vi "Alarm Flir-Ax8.vi"() -> ()   [LabVIEW 2016]
uses:
  <vilib>/sound2/lvsound2.llb/Sampling Mode.ctl
  <vilib>/sound2/lvsound2.llb/Sound File Info (path).vi
  <vilib>/sound2/lvsound2.llb/Sound File Read Open.vi
  Global Flir-Ax8.vi
  <vilib>/sound2/lvsound2.llb/Sound File Read (DBL).vi
  <vilib>/sound2/lvsound2.llb/Sound Output Write (DBL).vi
panel:
  in  "Number of Samples/Iteration":i32=2500
  in  "Device ID":u32
  out "Current Iteration":i32
  out "Current Data":waveform(dbl)[](graph)
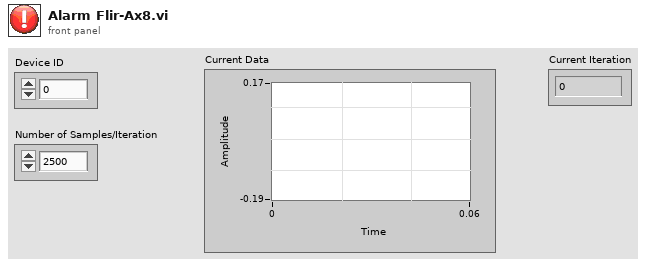
[diagram p1: front panel]
types:
  T1 = typedef "Sampling Mode.ctl" = i32
  T2 = typedef "Sound Data Format.ctl" = cluster{"sample rate (S/s)":dbl, "number of channels":i32, "bits per sample":i32}
  T3 = typedef "Sound File Refnum.ctl" = refnum<file>
  T4 = typedef "Sound Output Task ID.ctl" = u32
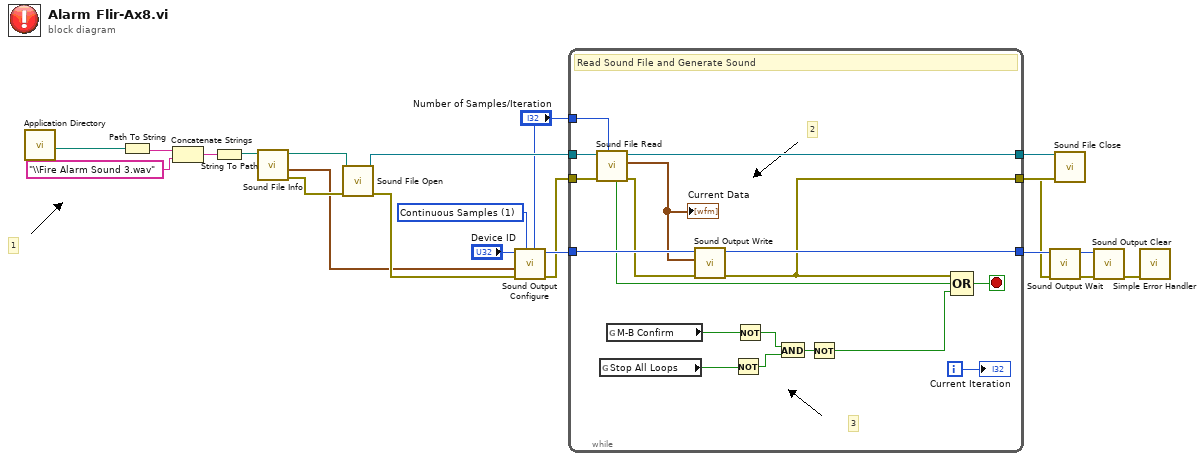
[diagram p0: block diagram]
diagram:
  w7 = T1 1 items=["Finite Samples", "Continuous Samples"] ("sample mode")
  # "1"
  n1 = call <vilib>:"Application Directory.vi"() -> ("Application Directory"=w2:path)
  n2 = Path To String(path=w2) -> (string=w4:string)
  n3 = Concatenate Strings ("add")(w4, "\\Fire Alarm Sound 3.wav" ("string")) -> (w5:string)
  n4 = String To Path(string=w5) -> (path=w1:path)
  n5 = call-poly <vilib>:"Sound File Info.vi"("path"=w1) -> ("error out"=w17:errorcluster, "sound format"=w9:T2, "path out"=w10:path)  [unwired: 7 in, 1 out]
  n6 = call-poly <vilib>:"Sound File Open.vi"("error in (no error)"=w17, "path"=w10) -> ("error out"=w16:errorcluster, "sound file refnum"=w18:T3)  [unwired: 8 in]
  n7 = call <vilib>:"Sound Output Configure.vi"("number of samples/ch"="Number of Samples/Iteration", "sample mode"=w7, "error in (no error)"=w16, "sound format"=w9, "device ID"="Device ID") -> ("error out"=w15:errorcluster, "task ID"=w22:T4)  [unwired: 5 in]
  n8 = while {
    tunnel: "Number of Samples/Iteration" -> [w31]
    tunnel: w18 -> [w38]
    tunnel: [w36] -> w20
    tunnel: w15 -> [w39]
    tunnel: [w30] -> w19
    tunnel: w22 -> [w35]
    tunnel: [w40] -> w13
    i -> [w37]
    stop <- w32 stop-if-true
    # "3"
    # "2"
    # "Read Sound File and Generate Sound"
    n9 = call-poly <vilib>:"Sound File Read.vi"("number of samples/ch (-1: all)"=w31, "error in (no error)"=w39, "sound file refnum"=w38) -> ("error out"=w34:errorcluster, "data"=w29:waveform(dbl)[], "sound file refnum out"=w36:T3, "end of file?"=w33:bool)  [unwired: 4 in, 1 out]
    "Current Data" <- w29
    n10 = global read "Global Flir-Ax8.vi" "Stop All Loops"() -> (w24:bool)
    n11 = global read "Global Flir-Ax8.vi" "M-B Confirm"() -> (w23:bool)
    n12 = call-poly <vilib>:"Sound Output Write.vi"("error in (no error)"=w34, "data"=w29, "task ID"=w35) -> ("error out"=w30:errorcluster, "task ID out"=w40:T4)  [unwired: 7 in]
    n13 = Not(x=w24) -> (.not. x?=w26:bool)
    n14 = Not(x=w23) -> (.not. x?=w27:bool)
    n15 = And(x=w27, y=w26) -> (x .and. y?=w25:bool)
    n16 = Not(x=w25) -> (.not. x?=w28:bool)
    n17 = Compound Arithmetic op=OR(w30, w33, w28) -> (w32:bool)
    "Current Iteration" <- w37
  }
  n18 = call <vilib>:"Sound File Close.vi"("error in (no error)"=w19, "sound file refnum"=w20) -> ("error out"=w12:errorcluster)  [unwired: 9 in]
  n19 = call <vilib>:"Sound Output Wait.vi"("error in (no error)"=w12, "task ID"=w13) -> ("error out"=w11:errorcluster, "task ID out"=w14:T4)  [unwired: 8 in]
  n20 = call <vilib>:"Sound Output Clear.vi"("error in (no error)"=w11, "task ID"=w14) -> ("error out"=w6:errorcluster)  [unwired: 9 in]
  n21 = call <vilib>:"Simple Error Handler.vi"("error in (no error)"=w6) -> ()  [unwired: 4 in, 5 out]
